vi "DMM_DC-RMS Current Meas Format Function Range.vi"(0 "DMM Handle In":refnum<k15>, 5 "Function Settings In":T4={"Range and Function"=enum."DC Current Auto Range", "Resolution in Digits"=5.5} {"Resolution in Digits" items=["3 1/2"=3.5, "4 1/2"=4.5, "5 1/2"=5.5, "6 1/2"=6.5, "7 1/2"=7.5]}, 11 "error in":errorcluster) -> (4 "DMM Handle Out":refnum<k15>, 6 "Function Settings Out":T3={"Range"=0.0, "Function"=enum."DC Volts", "Freq_Period AC Range"=0.0, "Resolution in Digits"=5.5} {"Resolution in Digits" items=["3 1/2"=3.5, "4 1/2"=4.5, "5 1/2"=5.5, "6 1/2"=6.5, "7 1/2"=7.5]}, 15 "error out":errorcluster)   [LabVIEW 2021, in "DMM_DC-RMS Current Measurement.lvlib"]
doc: "Utilizes the function settings input to select the particular function and range used for the measurement and format the output string displayed in the measurement output cluster."
uses:
  DMM_DC-RMS Current Measurement.lvlib
  Typedefs/Function Settings.ctl
  <instrlib>/niDMM/nidmm.llb/niDMM Resolution in Digits.ctl
  <instrlib>/niDMM/nidmm.llb/niDMM Function.ctl
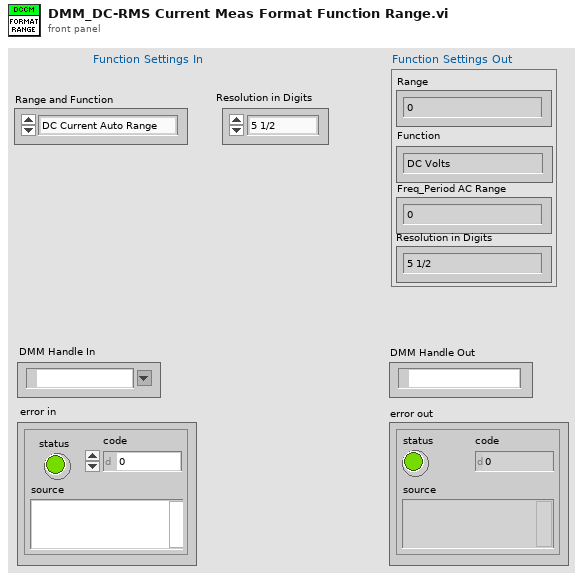
[diagram p1: front panel]
types:
  T1 = typedef "niDMM Function.ctl" = enum16{"DC Volts", "AC Volts", "DC Current", "AC Current", "2-wire Resistance", "4-wire Resistance", "Diode", "Frequency", "Period", "AC Volts DC Coupled", "Capacitance", "Inductance", "Temperature"}
  T2 = typedef "niDMM Resolution in Digits.ctl" = dbl
  T3 = cluster{"Range":dbl, "Function":T1, "Freq_Period AC Range":dbl, "Resolution in Digits":T2}
  T4 = typedef "DMM_DC-RMS Current Measurement.lvlib/Function Settings.ctl" = cluster{"Range and Function":enum16{"DC Current Auto Range", "DC 1 uA", "DC 10 uA", "DC 100 uA", "DC 1 mA", "DC 10 mA", "DC 20 mA", "DC 100 mA", "DC 200 mA", "DC 1 A", "DC 3 A", "   ", "AC Current Auto Range", "AC 100 uA", "AC 1 mA", "AC 10 mA", "AC 100 mA", "AC 500 mA", "AC 1 A", "AC 3 A"}, "Resolution in Digits":T2}
  T5 = enum16{"DC Current Auto Range", "DC 1 uA", "DC 10 uA", "DC 100 uA", "DC 1 mA", "DC 10 mA", "DC 20 mA", "DC 100 mA", "DC 200 mA", "DC 1 A", "DC 3 A", "   ", "AC Current Auto Range", "AC 100 uA", "AC 1 mA", "AC 10 mA", "AC 100 mA", "AC 500 mA", "AC 1 A", "AC 3 A"}
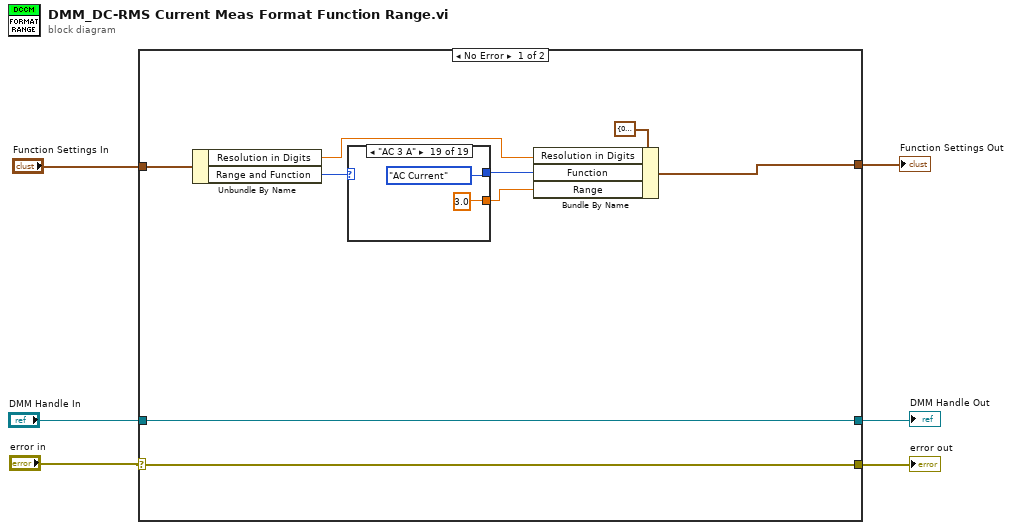
[diagram p0: block diagram]
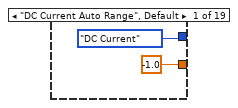
[diagram p2: hidden frame]
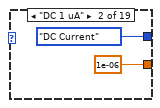
[diagram p3: hidden frame]
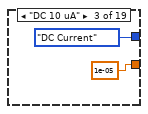
[diagram p4: hidden frame]
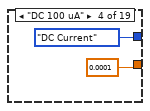
[diagram p5: hidden frame]
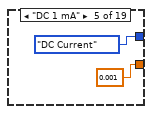
[diagram p6: hidden frame]
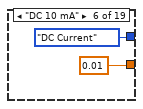
[diagram p7: hidden frame]
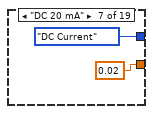
[diagram p8: hidden frame]
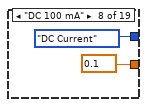
[diagram p9: hidden frame]
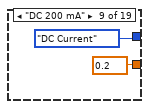
[diagram p10: hidden frame]
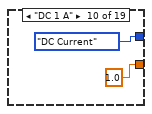
[diagram p11: hidden frame]
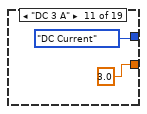
[diagram p12: hidden frame]
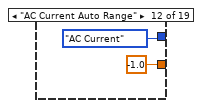
[diagram p13: hidden frame]
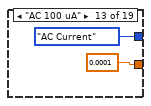
[diagram p14: hidden frame]
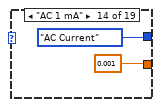
[diagram p15: hidden frame]
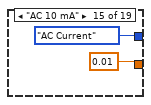
[diagram p16: hidden frame]
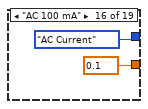
[diagram p17: hidden frame]
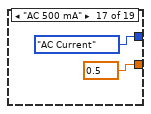
[diagram p18: hidden frame]
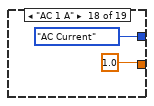
[diagram p19: hidden frame]
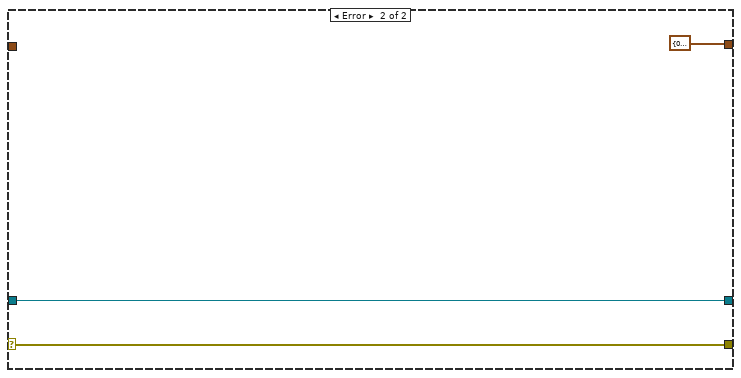
[diagram p20: hidden frame]
diagram:
  n1 = case shown="No Error" "error in" {
    selector: "error in" -> [w13 w55]
    tunnel: "Function Settings In" -> [w15 _]
    tunnel: [w9 T3 {"Range"=0.0, "Function"=enum."DC Volts", "Freq_Period AC Range"=0.0, "Resolution in Digits"=5.5} ("Function Settings Out")] -> w1
    tunnel: [w13 w55] -> w5
    tunnel: [w12 w56] -> w3
    tunnel: "DMM Handle In" -> [w12 w56]
    frame No Error {
      n2 = Unbundle By Name(w15) -> ("Resolution in Digits"=w14:T2, "Range and Function"=w11:T5)
      n3 = case shown="\"AC 3 A\"" w11 {
        tunnel: [niDMM_Function."DC Current" ("Function") niDMM_Function."DC Current" ("Function") niDMM_Function."DC Current" ("Function") niDMM_Function."DC Current" ("Function") niDMM_Function."DC Current" ("Function") niDMM_Function."DC Current" ("Function") niDMM_Function."DC Current" ("Function") niDMM_Function."DC Current" ("Function") niDMM_Function."DC Current" ("Function") niDMM_Function."DC Current" ("Function") niDMM_Function."DC Current" ("Function") niDMM_Function."AC Current" ("Function") niDMM_Function."AC Current" ("Function") niDMM_Function."AC Current" ("Function") niDMM_Function."AC Current" ("Function") niDMM_Function."AC Current" ("Function") niDMM_Function."AC Current" ("Function") niDMM_Function."AC Current" ("Function") niDMM_Function."AC Current" ("Function")] -> w7
        tunnel: [-1.0 ("Range") 1e-06 ("Range") 1e-05 ("Range") 0.0001 ("Range") 0.001 ("Range") 0.01 ("Range") 0.02 ("Range") 0.1 ("Range") 0.2 ("Range") 1.0 ("Range") 3.0 ("Range") -1.0 ("Range") 0.0001 ("Range") 0.001 ("Range") 0.01 ("Range") 0.1 ("Range") 0.5 ("Range") 1.0 ("Range") 3.0 ("Range")] -> w8
        frame "DC Current Auto Range", Default {
        }
        frame "DC 1 uA" {
        }
        frame "DC 10 uA" {
        }
        frame "DC 100 uA" {
        }
        frame "DC 1 mA" {
        }
        frame "DC 10 mA" {
        }
        frame "DC 20 mA" {
        }
        frame "DC 100 mA" {
        }
        frame "DC 200 mA" {
        }
        frame "DC 1 A" {
        }
        frame "DC 3 A" {
        }
        frame "AC Current Auto Range" {
        }
        frame "AC 100 uA" {
        }
        frame "AC 1 mA" {
        }
        frame "AC 10 mA" {
        }
        frame "AC 100 mA" {
        }
        frame "AC 500 mA" {
        }
        frame "AC 1 A" {
        }
        frame "AC 3 A" {
        }
      }
      n4 = Bundle By Name(cluster=T3 {"Range"=0.0, "Function"=enum."DC Volts", "Freq_Period AC Range"=0.0, "Resolution in Digits"=5.5} ("Function Settings Out"), "Resolution in Digits"=w14, "Function"=w7, "Range"=w8) -> (w9:T3)
    }
    frame Error {
    }
  }
  "error out" <- w5
  "DMM Handle Out" <- w3
  "Function Settings Out" <- w1
